vi "Scale FP Controls.vi"(8 "error in (no error)":errorcluster, 10 "Pane":refnum<vi>, 11 "AppMgr in":refnum<class "Application Manager.lvclass">) -> (0 "error out":errorcluster, 3 "AppMgr out":refnum<class "Application Manager.lvclass">)   [LabVIEW 2017, in "Application Manager.lvclass"]
doc: "Resize resizable front panel elements"
uses:
  Application Manager.lvclass
  Application Manager.lvclass/Application Manager.ctl
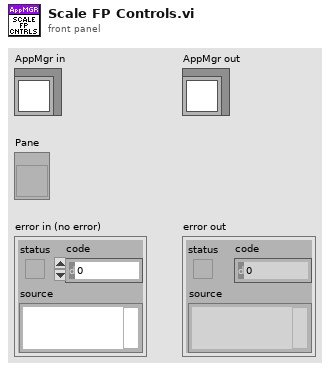
[diagram p1: front panel]
types:
  T1 = typedef "LVPositionTypeDef.ctl" = cluster{"Left":i32, "Top":i32}
  T2 = typedef "LVBoundsTypeDef.ctl" = cluster{"Width":u32, "Height":u32}
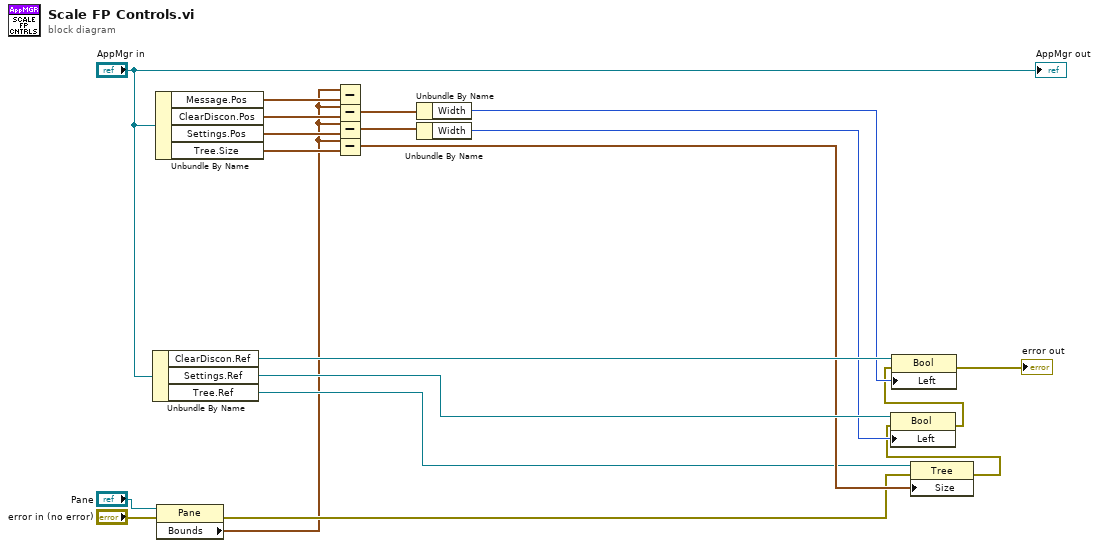
[diagram p0: block diagram]
diagram:
  n1 = Unbundle By Name("AppMgr in") -> ("ClearDiscon.Ref"=w13:refnum<vi>, "Settings.Ref"=w8:refnum<vi>, "Tree.Ref"=w3:refnum<vi>)
  n2 = Unbundle By Name("AppMgr in") -> ("Message.Pos"=w18:T1, "ClearDiscon.Pos"=w15:T1, "Settings.Pos"=w16:T1, "Tree.Size"=w17:T2)
  n3 = property class="Pane"(reference="Pane", error in="error in (no error)") -> (error out=w4:errorcluster, "Bounds"=w1:T2)  [unwired: 1 out]
  n4 = Subtract(x=w1, y=w18) -> ()  [unwired: 1 out]
  n5 = Subtract(x=w1, y=w15) -> (x-y=w14:T2)
  n6 = Subtract(x=w1, y=w16) -> (x-y=w11:T2)
  n7 = Subtract(x=w1, y=w17) -> (x-y=w5:T2)
  n8 = Unbundle By Name(w14) -> ("Width"=w12:u32)
  n9 = Unbundle By Name(w11) -> ("Width"=w7:u32)
  n10 = property class="Tree"(reference=w3, error in=w4, "Size"=w5) -> (error out=w6:errorcluster)  [unwired: 1 out]
  n11 = property class="Bool"(reference=w8, error in=w6, "Left"=w7) -> (error out=w9:errorcluster)  [unwired: 1 out]
  n12 = property class="Bool"(reference=w13, error in=w9, "Left"=w12) -> (error out=→"error out":errorcluster)  [unwired: 1 out]
  "AppMgr out" <- "AppMgr in"
